vi "main.vi"() -> ()   [LabVIEW 2021]
uses:
  <vilib>/OPCUA/controls/NodeId.ctl
  <vilib>/OPCUA/NI OPC UA Client.lvlib
panel:
  in  "Distant Control":bool
  in  "Distant Control from OPC":bool
  in  "Simulation":bool
  out "DISTANT_CONTROL_ENABLE":bool
  out "DISTANT_CONTROL_TALKBACK":bool
  out "DISTANT_CONTROL_AERPUMP":bool=TRUE
  in  "Server endpoint URL":string="opc.tcp://localhost:4840/"
  out "DISTANT_CONTROL_WATCHDOG":i32
  in  "Oxygen concentration":dbl(slide) scale=1.5..2.5
  in  "Stop":bool
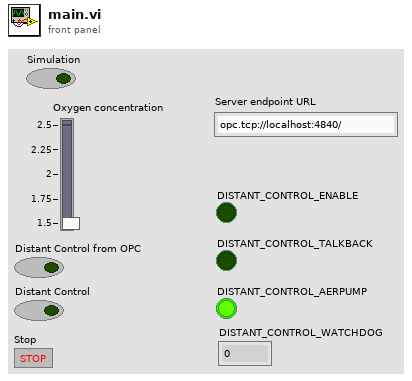
[diagram p1: front panel]
types:
  T1 = typedef "NodeId.ctl" = string
  T2 = typedef "OPC UA Client Refnum.ctl" = refnum<k21>
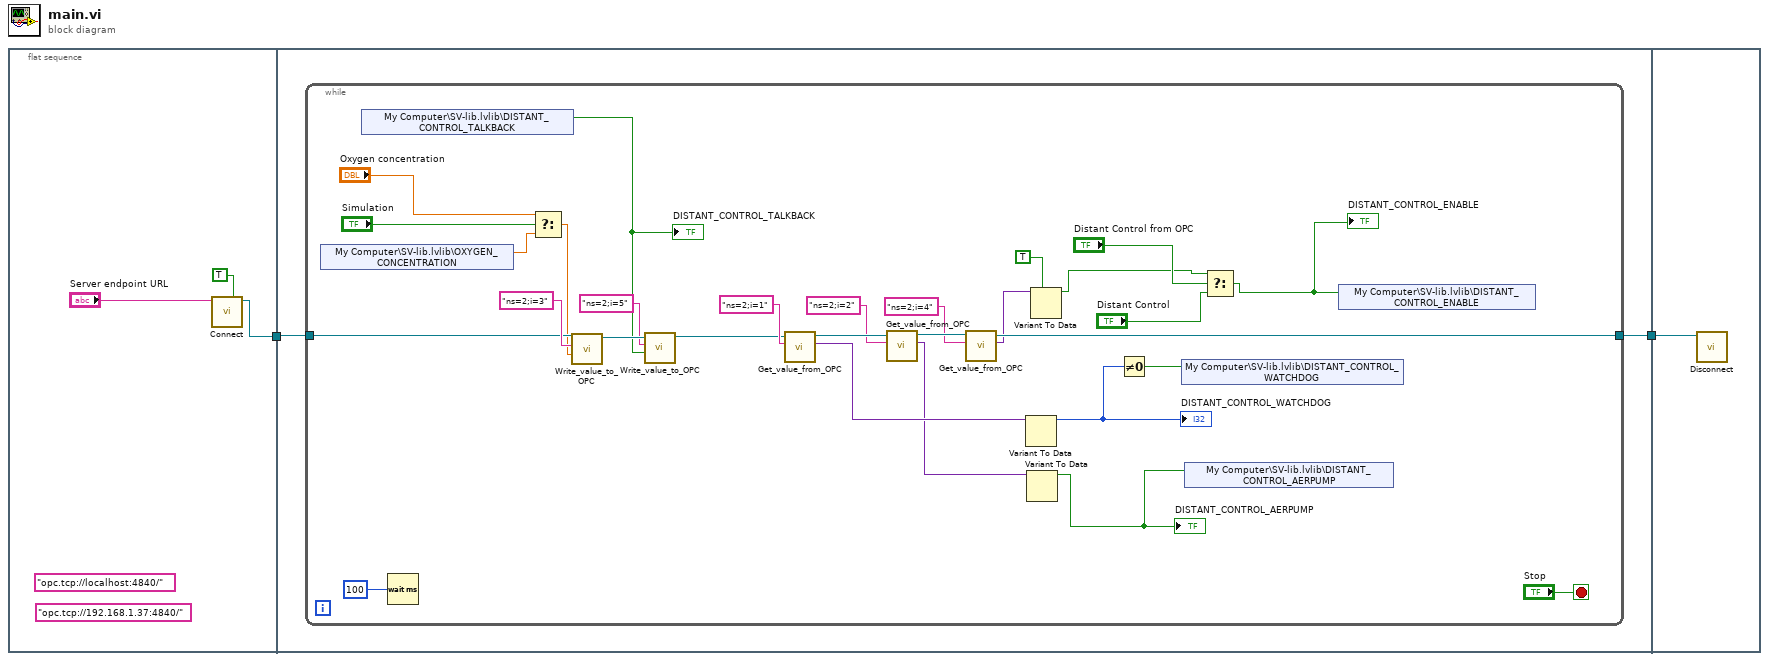
[diagram p0: block diagram]
diagram:
  n1 = flat-sequence {
    tunnel: [w4] -> w2
    tunnel: w2 -> [w7]
    tunnel: [w6] -> w1
    tunnel: w1 -> [w37]
    frame #0 {
      (unwired) "opc.tcp://192.168.1.37:4840/" ("server endpoint URL")
      (unwired) "opc.tcp://localhost:4840/" ("server endpoint URL")
      n2 = call <vilib>:"Connect.vi"("trust any server (F)"=TRUE, "server endpoint URL"="Server endpoint URL") -> ("OPC UA client refnum out"=w4:T2)  [unwired: 7 in, 2 out]
    }
    frame #1 {
      n3 = while {
        tunnel: w7 -> [w26]
        tunnel: [w21] -> w6
        stop <- "Stop" stop-if-true
        n4 = shared-variable "My Computer\\SV-lib.lvlib\\OXYGEN_CONCENTRATION"() -> (w13:dbl)  [unwired: 1 in, 1 out]
        n5 = shared-variable "My Computer\\SV-lib.lvlib\\DISTANT_CONTROL_TALKBACK"() -> (w16:bool)  [unwired: 1 in, 1 out]
        "DISTANT_CONTROL_TALKBACK" <- w16
        n6 = Wait (ms)(milliseconds to wait=u32 100) -> ()  [unwired: 1 out]
        n7 = Select(t="Oxygen concentration", s="Simulation", f=w13) -> (s? t:f=w12:dbl)
        n8 = call "Write_value_to_OPC.vi"("Data in"=w12, "Address to write"=T1 "ns=2;i=3" ("node ID"), "OPC UA client refnum in"=w26) -> ("OPC UA client refnum out"=w24:T2)  [unwired: 8 in]
        n9 = call "Write_value_to_OPC.vi"("Data in"=w16, "Address to write"=T1 "ns=2;i=5" ("node ID"), "OPC UA client refnum in"=w24) -> ("OPC UA client refnum out"=w23:T2)  [unwired: 8 in]
        n10 = call "Get_value_from_OPC.vi"("Address to read"=T1 "ns=2;i=1" ("node ID"), "OPC UA client refnum in"=w23) -> ("Data out"=w31:variant, "OPC UA client refnum out"=w34:T2)  [unwired: 5 in, 1 out]
        n11 = call "Get_value_from_OPC.vi"("Address to read"=T1 "ns=2;i=2" ("node ID"), "OPC UA client refnum in"=w34) -> ("Data out"=w30:variant, "OPC UA client refnum out"=w25:T2)  [unwired: 5 in, 1 out]
        n12 = call "Get_value_from_OPC.vi"("Address to read"=T1 "ns=2;i=4" ("node ID"), "OPC UA client refnum in"=w25) -> ("Data out"=w19:variant, "OPC UA client refnum out"=w21:T2)  [unwired: 5 in, 1 out]
        n13 = Variant To Data(Variant=w31) -> (data=w17:i32)  [unwired: 2 in, 1 out]
        "DISTANT_CONTROL_WATCHDOG" <- w17
        n14 = Variant To Data(Variant=w30) -> (data=w28:bool)  [unwired: 2 in, 1 out]
        "DISTANT_CONTROL_AERPUMP" <- w28
        n15 = Variant To Data(type=TRUE, Variant=w19) -> (data=w9:bool)  [unwired: 1 in, 1 out]
        n16 = Not Equal To 0?(x=w17) -> (x != 0?=w27:bool)
        n17 = shared-variable "My Computer\\SV-lib.lvlib\\DISTANT_CONTROL_WATCHDOG"(w27) -> ()  [unwired: 1 in, 1 out]
        n18 = shared-variable "My Computer\\SV-lib.lvlib\\DISTANT_CONTROL_AERPUMP"(w28) -> ()  [unwired: 1 in, 1 out]
        n19 = Select(t=w9, s="Distant Control from OPC", f="Distant Control") -> (s? t:f=w8:bool)
        "DISTANT_CONTROL_ENABLE" <- w8
        n20 = shared-variable "My Computer\\SV-lib.lvlib\\DISTANT_CONTROL_ENABLE"(w8) -> ()  [unwired: 1 in, 1 out]
      }
    }
    frame #2 {
      n21 = call <vilib>:"Disconnect.vi"("OPC UA client refnum in"=w37) -> ()  [unwired: 10 in, 1 out]
    }
  }
